vi "Process Job.vi"(8 "error in":errorcluster, 10 "Task":refnum<class>, 11 "Worker in":refnum<class "Worker.lvclass">) -> (0 "error out":errorcluster, 3 "Worker out":refnum<class "Worker.lvclass">)   [LabVIEW 2023, in "Worker.lvlib" / "Worker.lvclass"]
doc: "Perform the task assigned by the work dispatcher. This method is required by any descendant of the Worker class."
uses:
  Worker.lvclass
  c:/dev/_r/4/eng/lv-core/lvpostprocessingd/lv_mc_x86_64/dist_i386/vi.lib/ActorFramework/Actor/Actor.lvclass
  <vilib>/ActorFramework/Actor/Actor.lvclass/Actor.ctl
  <vilib>/ActorFramework/Message Enqueuer/Message Enqueuer.lvclass/Message Enqueuer.ctl
  Person Messages/Increase Count Msg/Increase Count Msg.lvclass/Increase Count Msg.ctl
  <vilib>/ActorFramework/Message Enqueuer/Init from Existing Queue.vi
  <vilib>/ActorFramework/Message Enqueuer/Enqueue.vi
  Person Messages/Increase Count Msg/Increase Count Msg.lvclass
  c:/dev/_r/4/eng/lv-core/lvpostprocessingd/lv_mc_x86_64/dist_i386/vi.lib/ActorFramework/Message/Message.lvclass
  <vilib>/ActorFramework/Message Priority Queue/Priority Enqueue.vi
  <vilib>/ActorFramework/Message Enqueuer/Message Enqueuer.lvclass
  <vilib>/ActorFramework/Actor/Actor.lvclass
panel:
  in  "Waiting":string="Waiting..."
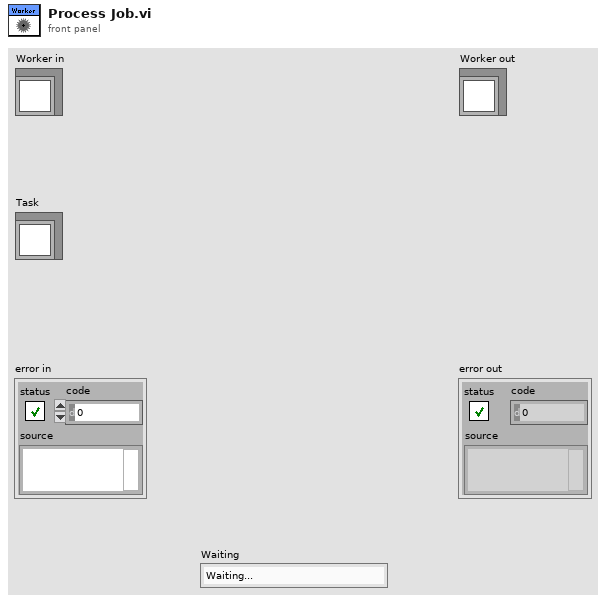
[diagram p1: front panel]
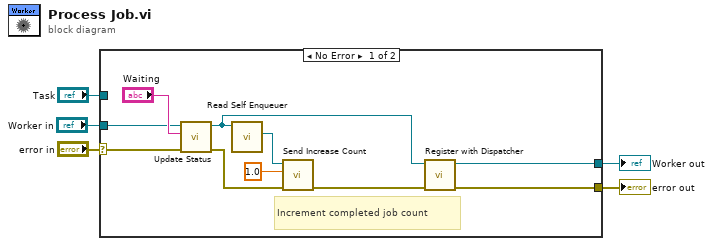
[diagram p0: block diagram]
diagram:
  n1 = case shown="No Error" "error in" {
    selector: "error in" -> [w12 w17]
    tunnel: [w14 w17] -> w4
    tunnel: [w6 w16] -> w2
    tunnel: "Worker in" -> [w10 w16]
    tunnel: "Task" -> [_ _]
    frame No Error {
      # "Increment completed job count"
      n2 = call-dynamic "Update Status.vi"("error in (no error)"=w12, "Status"="Waiting", "Worker in"=w10) -> ("error out"=w11:errorcluster, "Worker out"=w7:refnum<class "Worker.lvclass">)  [unwired: 7 in]
      n3 = call <vilib>:"Read Self Enqueuer.vi"("Actor"=w7) -> ("Self Enqueuer"=w15:refnum<class "Message Enqueuer.lvclass">)  [unwired: 10 in]
      n4 = call "Send Increase Count.vi"("error in (no error)"=w11, "Amount"=1.0, "Message Enqueuer"=w15) -> ("error out"=w8:errorcluster)  [unwired: 7 in, 1 out]
      n5 = call-dynamic "Register with Dispatcher.vi"("error in (no error)"=w8, "Worker in"=w7) -> ("error out"=w14:errorcluster, "Worker out"=w6:refnum<class "Worker.lvclass">)  [unwired: 8 in]
    }
    frame Error {
    }
  }
  "error out" <- w4
  "Worker out" <- w2
